vi "Password.vi"(1 "Password In":string) -> (0 "Password out":string)   [LabVIEW 2020]
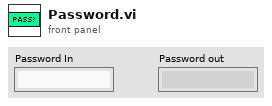
[diagram p1: front panel]
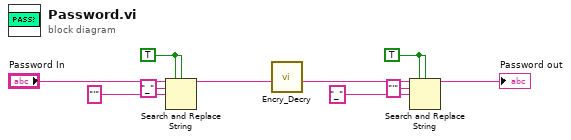
[diagram p0: block diagram]
diagram:
  w6 = TRUE ("replace all? (F)")
  w7 = TRUE ("replace all? (F)")
  n1 = Search and Replace String(replace all?=w6, case sensitive?=w6, input string="Password In", search string="_", replace string="'" ("replace string (\"\")")) -> (result string=w2:string)  [unwired: 3 in, 3 out]
  n2 = call <userlib>:"Encry_Decry.vi"("Password in"=w2) -> ("Password out"=w8:string)  [unwired: 10 in]
  n3 = Search and Replace String(replace all?=w7, case sensitive?=w7, input string=w8, search string="'", replace string="_" ("replace string (\"\")")) -> (result string=→"Password out":string)  [unwired: 3 in, 3 out]
